vi "ENPH 354 Assignment 3 - Q2.vi"() -> ()   [LabVIEW 2021]
panel:
  in  "?":bool
  out "Waveform Chart":dbl(graph)
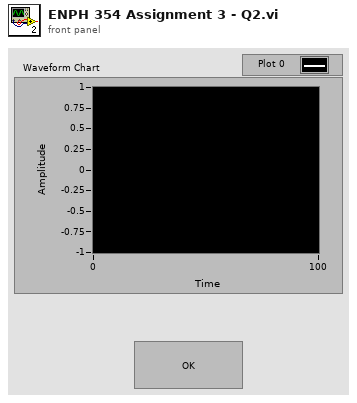
[diagram p1: front panel]
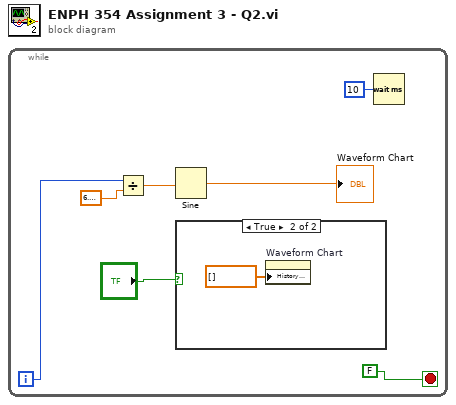
[diagram p0: block diagram]
diagram:
  n1 = while {
    i -> [w7]
    stop <- FALSE stop-if-true
    n2 = Divide(x=w7, y=6.283185307179586) -> (x/y=w5:dbl)
    n3 = Sine(x=w5) -> (sin(x)=→"Waveform Chart":dbl)
    n4 = case shown="True" "?" {
      frame False {
      }
      frame True {
        n5 = property on="Waveform Chart" class="WFChart (strict)"("History Data"=dbl[] []) -> ()  [unwired: 2 in, 2 out]
      }
    }
    n6 = Wait (ms)(milliseconds to wait=u32 10) -> ()  [unwired: 1 out]
  }
